vi "sendValue.vi"(8 "error in (no error)":errorcluster, 10 "data":variant, 11 "azimuthInPosition in":refnum<class "azimuthInPosition.lvclass">) -> (0 "error out":errorcluster, 2 "function return":i32, 3 "azimuthInPosition out":refnum<class "azimuthInPosition.lvclass">)   [LabVIEW 2016, in "SALLV_AtDome_Messaging.lvlib" / "azimuthInPosition.lvclass"]
uses:
  azimuthInPosition.lvclass
  ts_sallv_AtDome/DataTypes/logevent_azimuthInPosition.ctl
  ts_sallv_AtDome/SALLV_AtDome.lvlib
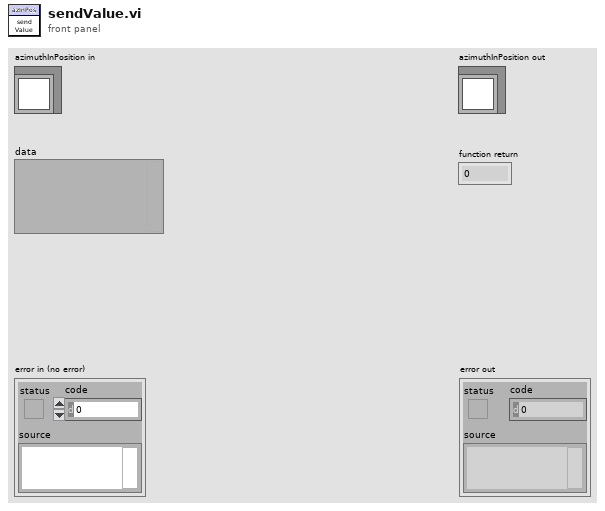
[diagram p1: front panel]
types:
  T1 = typedef "SALLV_AtDome.lvlib/logevent_azimuthInPosition.ctl" = cluster{"inPosition":bool, "priority":i32}
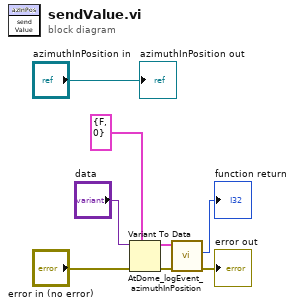
[diagram p0: block diagram]
diagram:
  n1 = Variant To Data(error in="error in (no error)", type=T1 {"inPosition"=FALSE, "priority"=0} ("logevent_azimuthInPosition_Ctl"), Variant="data") -> (data=w5:T1, error out=w4:errorcluster)
  n2 = call "AtDome_logEvent_azimuthInPosition.vi"("error in (no error)"=w4, "logevent_azimuthInPosition_Ctl"=w5) -> ("error out"=→"error out":errorcluster, "function return"=→"function return":i32)  [unwired: 7 in, 1 out]
  "azimuthInPosition out" <- "azimuthInPosition in"
